vi "C to F.vi"() -> ()   [LabVIEW 2023]
doc: "Ersteller: Sara\nDatum: 21.11.2025\n\nKurzbeschreibung:\nDieses SubVI rechnet zwischen °C und °F um.\n\nTRUE = Celsius ? Fahrenheit\nFALSE = Fahrenheit ? Celsius\n\nEingänge:\n- Input Temperature (numeric)\n- C to F? (boolean)\n\nAusgang:\n- Output Temperature (numeric)"
panel:
  out "Output Temperature":dbl
  in  "C to F?":bool
  in  "Input Temperature":dbl
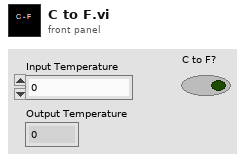
[diagram p1: front panel]
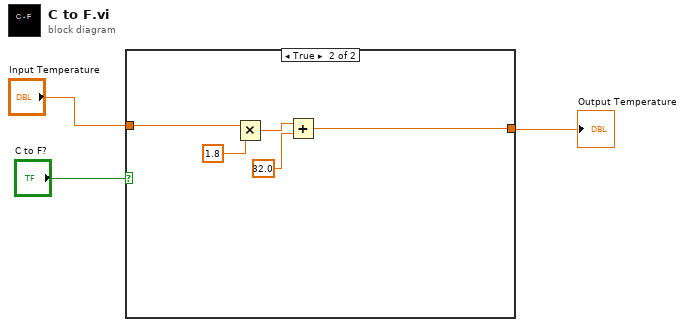
[diagram p0: block diagram]
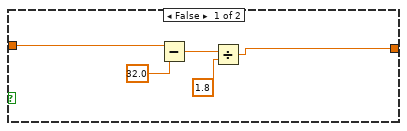
[diagram p2: hidden frame]
diagram:
  n1 = case shown="True" "C to F?" {
    tunnel: [w4 w10] -> w1
    tunnel: "Input Temperature" -> [w5 w9]
    frame False {
      n2 = Subtract(x=w5, y=32.0) -> (x-y=w7:dbl)
      n3 = Divide(x=w7, y=1.8) -> (x/y=w4:dbl)
    }
    frame True {
      n4 = Multiply(x=w9, y=1.8) -> (x*y=w12:dbl)
      n5 = Add(x=w12, y=32.0) -> (x+y=w10:dbl)
    }
  }
  "Output Temperature" <- w1
